vi "_getBinFileContents.vi"(8 "error in":errorcluster, 10 "binFile":path) -> (0 "error out":errorcluster, 4 "chunkedData":u8[][](array[numeric]), 5 "numUpdates":i32, 6 "data":u8[](array[numeric]) format="%.0x", 7 "numBytes":i64)   [LabVIEW 2017]
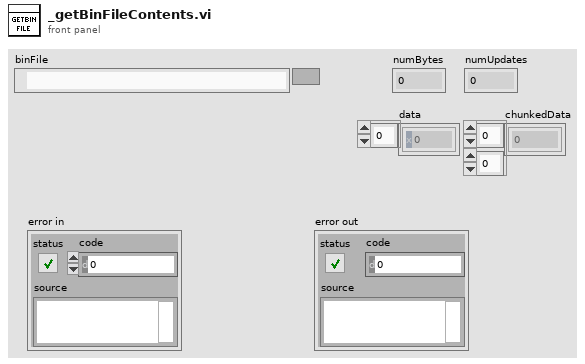
[diagram p1: front panel]
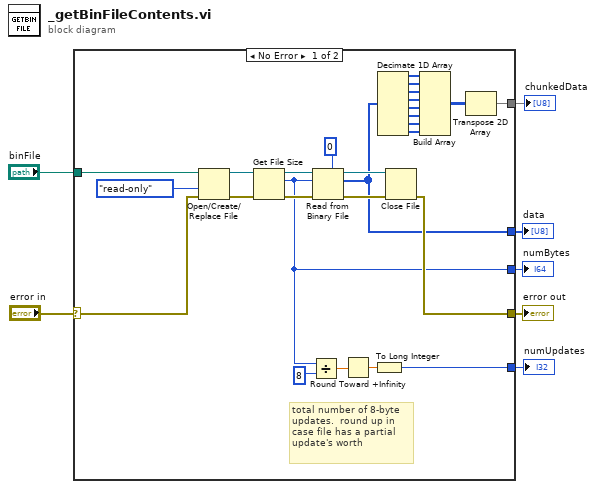
[diagram p0: block diagram]
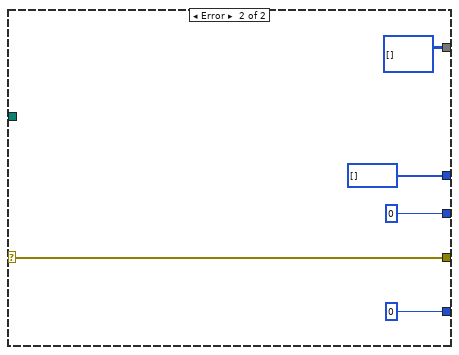
[diagram p2: hidden frame]
diagram:
  n1 = case shown="No Error" "error in" {
    selector: "error in" -> [w25 w39]
    tunnel: "binFile" -> [w33 _]
    tunnel: [w18 u8[] []] -> w6
    tunnel: [w22 i64 0 ("size (in bytes)")] -> w5
    tunnel: [w24 w39] -> w3
    tunnel: [w19 0] -> w2
    tunnel: [w8 u8[][] []] -> w1
    frame No Error {
      # "total number of 8-byte\nupdates.  round up in \ncase file has a partial\nupdate's worth"
      n2 = Open/Create/Replace File(file path (use dialog)=w33, error in=w25, access (0:read/write)=enum16{"read/write", "read-only", "write-only"}."read-only") -> (refnum out=w32:refnum<file>, error out=w31:errorcluster)  [unwired: 3 in, 1 out]
      n3 = Get File Size(file=w32, error in=w31) -> (refnum out=w29:refnum<file>, size (in bytes)=w22:i64, 0:w30:errorcluster)
      n4 = Divide(x=w22, y=i64 8) -> (x/y=w23:dbl)
      n5 = Read from Binary File(5:u8 0, 8:w30, 10:w22, 11:w29) -> (0:w28:errorcluster, 2:w18:u8[], 3:w27:refnum<file>)  [unwired: 2 in, 1 out]
      n6 = Round Toward +Infinity(x=w23) -> (ceil(x): smallest int >= x=w20:dbl)
      n7 = To Long Integer(number=w20) -> (32bit integer=w19:i32)
      n8 = Decimate 1D Array(w18) -> (w17:u8[], w16:u8[], w15:u8[], w14:u8[], w13:u8[], w12:u8[], w11:u8[], w10:u8[])
      n9 = Close File(refnum=w27, error in=w28) -> (error out=w24:errorcluster)  [unwired: 1 out]
      n10 = Build Array(w17, w16, w15, w14, w13, w12, w11, w10) -> (w9:u8[][])
      n11 = Transpose 2D Array(2D array=w9) -> (transposed array=w8:u8[][])
    }
    frame Error {
    }
  }
  "data" <- w6
  "numBytes" <- w5
  "error out" <- w3
  "numUpdates" <- w2
  "chunkedData" <- w1
